vi "Curtin_CheckNewLoc.vi"(6 "Settings":T2={"Name of test"="", "Date"=timestamp(0 s since 1904-01-01), "Location"="", "Template"="", "Soundcard"="", "resolution"=32, "Sampling rate"=48000, "Ch1 Gain "=25.0, "Ch2 Gain"=10.0, "Sample time (s)"=0.3, "Pre-trigger (s)"=0.01, "Hammer Threshold"=10.0, "Positions"=12, "Taps/Position"=5, "Set Names"="", "Freq resolution"=10.0, "Hammer cutoff"=0.0, "Mic cutoff"=0.0, "Double bounce "=0.0, "Hammer Cal"=10.0, "dB Offset"=0.0, "Accel Cal"=10.0, "Vibrometer Cal"=0.0, "Mic Cal"=0.0, "Output"=2, "Voltage Cal"=1.0, "Vibrometer Port"="ASRL27::INSTR", "Range"=4, "High Pass"=2, "Bandwidth"=4, "X Range"=[], "Y Range"=[], "dB Spread"=0.0, "Trigger"=0, "Ch_1"=25, "Ch_2"=25, "flip?"=FALSE, "60Hz"=FALSE, "Time offset"=0.0, "Piezo Cal"=1.0, "Default Notes"=""} {"Ch_2" min=1 step=1; "Ch_1" min=1 max=100 step=1; "Trigger" items=["Hammer (force)", "Self-tap", "Spacebar"]; "Bandwidth" items=["1 kHz"=1, "5 kHz"=5, "10 kHz"=10, "25 kHz"=25, "50 kHz"=50, "100 kHz"=100]; "High Pass" items=["Off", "13 Hz", "104 Hz"]; "Range" items=["10 mm/s"=1, "20 mm/s"=2, "50 mm/s"=5, "100 mm/s"=10, "200 mm/s"=20, "500 mm/s"=50, "1 m/s"=100, "2 m/s"=200]; "Output" items=["Accelerometer", "Speed (from acceleration)", "Microphone", "Vibrometer", "Piezo"]; "Voltage Cal" format="%#_13g"; "Ch2 Gain" format="%#_13g"; "Ch1 Gain" format="%#_13g"; "Double bounce" min=0.0; "Mic cutoff" min=0.0 format="%#_4g"; "Hammer cutoff" min=0.0 format="%#_4g"; "Freq resolution" min=0.0; "Pre-trigger (s)" format="%#_13g"; "Date" format="%<%H:%M\n%d/%m/%y>T"; "resolution" items=["16 bit"=16, "24 bit"=24, "32 bit"=32]; "Sampling rate" items=["22050 samp/s"=22050, "44100 samp/s"=44100, "48000 samp/s"=48000]}, 8 "Last Data File":path, 11 "Alarms":refnum<vi>) -> (0 "Last Data Set":path, 1 "Task":T1(ring), 2 "Keep Set?":bool, 3 "Done?":bool, 4 "New Set":bool, 5 "Pause?":bool)   [LabVIEW 2022 SP3]
uses:
  PreferencesControl.ctl
  Mic_Global.vi
panel:
  # "Hz"
  # "dB"
  # "dB"
  # "sec"
  # "sec"
  # "mV/Pa"
  # "mV/m/s2"
  # "mV/mm/s"
  # "V/N"
  # "sec"
  # "sec"
  # "mV/N"
  # "a.u."
  # "a.u."
  # "sec"
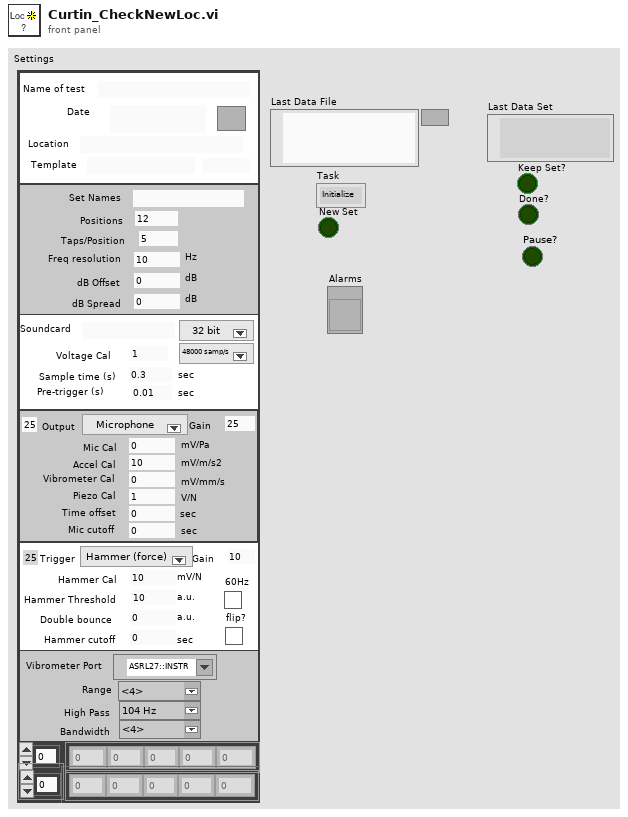
[diagram p1: front panel]
types:
  T1 = enum16{"Initialize", "Free run", "One Shot - waiting", "One Shot - triggered", "Wait", "Close"}
  T2 = typedef "PreferencesControl.ctl" = cluster{"Name of test":string, "Date":timestamp, "Location":string, "Template":string, "Soundcard":string, "resolution":u16, "Sampling rate":u16, "Ch1 Gain ":dbl, "Ch2 Gain":dbl, "Sample time (s)":dbl, "Pre-trigger (s)":dbl, "Hammer Threshold":dbl, "Positions":i16, "Taps/Position":i16, "Set Names":string, "Freq resolution":dbl, "Hammer cutoff":dbl, "Mic cutoff":dbl, "Double bounce ":dbl, "Hammer Cal":dbl, "dB Offset":dbl, "Accel Cal":dbl, "Vibrometer Cal":dbl, "Mic Cal":dbl, "Output":u16, "Voltage Cal":dbl, "Vibrometer Port":refnum<visa-resource-name>, "Range":u16, "High Pass":u16, "Bandwidth":u16, "X Range":cluster{"Minimum":dbl, "Maximum":dbl, "Increment":dbl, "Minor Increment":dbl, "Start":dbl}[], "Y Range":cluster{"Minimum":dbl, "Maximum":dbl, "Increment":dbl, "Minor Increment":dbl, "Start":dbl}[], "dB Spread":dbl, "Trigger":u16, "Ch_1":u8, "Ch_2":u8, "flip?":bool, "60Hz":bool, "Time offset":dbl, "Piezo Cal":dbl, "Default Notes":string}
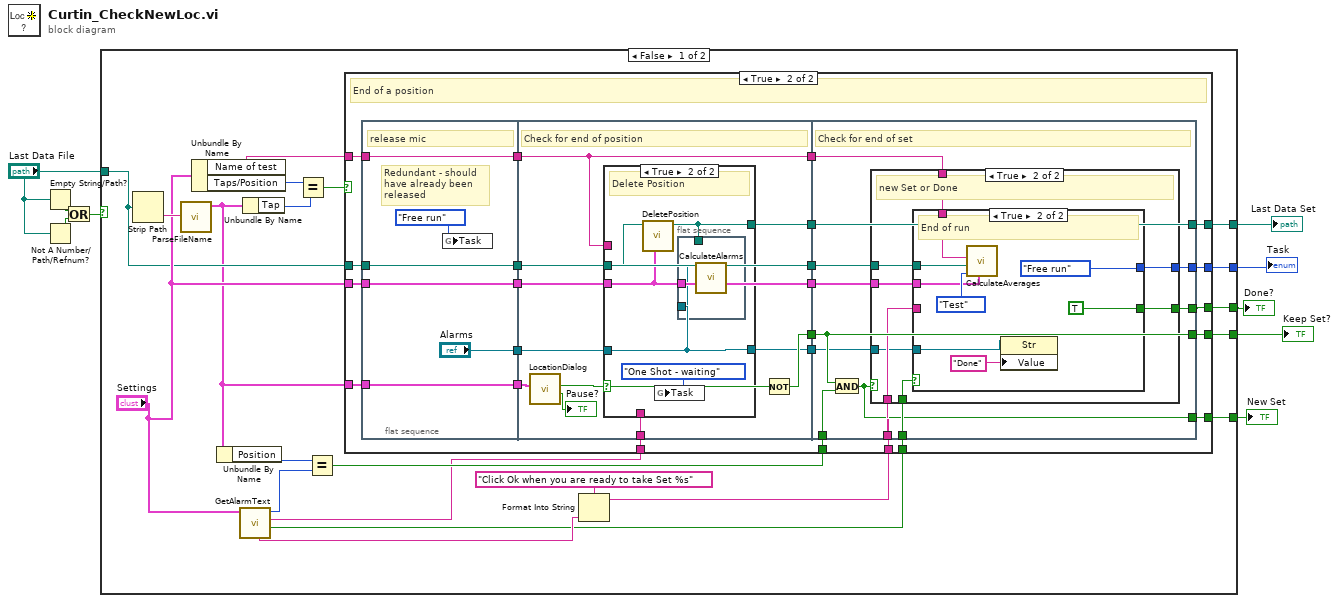
[diagram p0: block diagram]
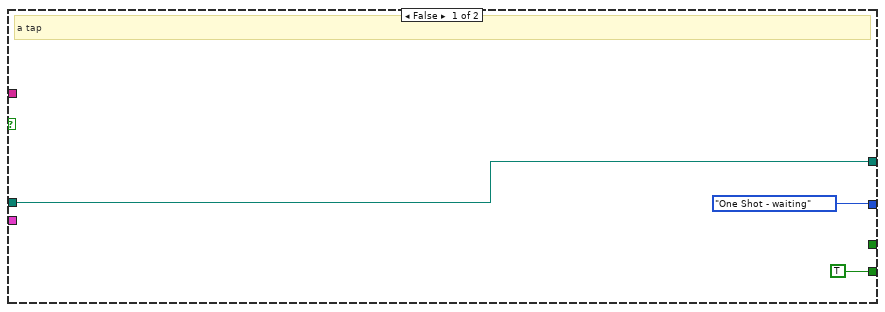
[diagram p2: hidden frame]
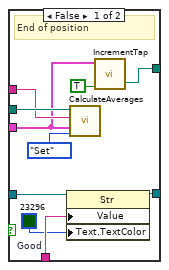
[diagram p3: hidden frame]
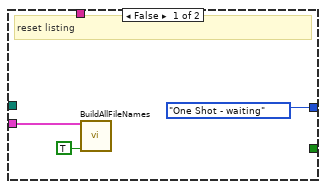
[diagram p4: hidden frame]
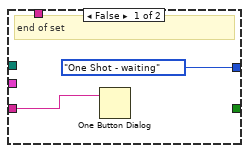
[diagram p5: hidden frame]
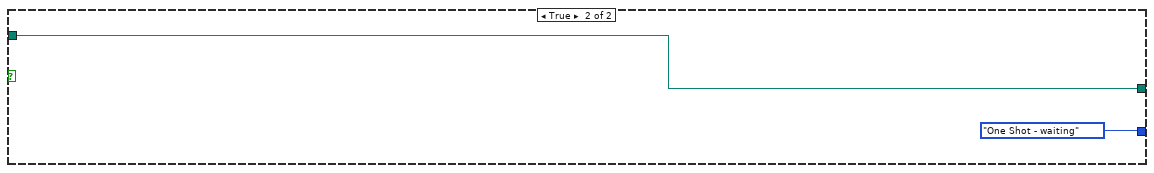
[diagram p6: hidden frame]
diagram:
  n1 = Empty String/Path?(string/path="Last Data File") -> (empty?=w5:bool)
  n2 = Not A Number/Path/Refnum?(number/path/refnum="Last Data File") -> (NaN/Path/Refnum?=w4:bool)
  n3 = Or(x=w5, y=w4) -> (x .or. y?=w3:bool)
  n4 = case shown="False" w3 {
    tunnel: [w23 _] -> w9
    tunnel: [w18 w126] -> w8
    tunnel: [w17 _] -> w7
    tunnel: "Last Data File" -> [w16 w126]
    tunnel: [w14 T1."One Shot - waiting" ("Task")] -> w2
    tunnel: [w13 _] -> w1
    frame False {
      n5 = Strip Path(path=w16) -> (name=w30:string)  [unwired: 1 out]
      n6 = call "ParseFileName.vi"("String in"=w30) -> ("Info"=w15:cluster{"Set":string, "Position":i32, "Tap":i32})  [unwired: 2 out]
      n7 = Unbundle By Name("Settings") -> ("Name of test"=w24:string, "Taps/Position"=w28:i16)
      n8 = Unbundle By Name(w15) -> ("Position"=w26:i32)
      n9 = call "GetAlarmText.vi"("Settings"="Settings") -> ("Done?"=w11:bool, "text"=w10:string, "Positions"=w27:i16, "Set Names"=w12:string)  [unwired: 7 in]
      n10 = Unbundle By Name(w15) -> ("Tap"=w29:i32)
      n11 = Equal?(x=w28, y=w29) -> (x = y?=w21:bool)
      n12 = Equal?(x=w26, y=w27) -> (x = y?=w25:bool)
      n13 = Format Into String(format string="Click Ok when you are ready to take Set %s" ("Text"), w12) -> (resulting string=w19:string)  [unwired: 2 in, 1 out]
      n14 = case shown="True" w21 {
        tunnel: w16 -> [w33 w57]
        tunnel: w19 -> [_ w55]
        tunnel: w25 -> [_ w54]
        tunnel: w11 -> [_ w53]
        tunnel: w24 -> [_ w45]
        tunnel: [_ w50] -> w23
        tunnel: "Settings" -> [_ w49]
        tunnel: [w33 w43] -> w18
        tunnel: [TRUE w41] -> w17
        tunnel: w15 -> [_ w40]
        tunnel: [T1."One Shot - waiting" ("Task") w38] -> w14
        tunnel: [_ w37] -> w13
        tunnel: w10 -> [_ w34]
        frame False {
          # "a tap"
        }
        frame True {
          # "End of a position"
          n15 = flat-sequence {
            tunnel: w57 -> [w62]
            tunnel: [w62] -> w56
            tunnel: w49 -> [w61]
            tunnel: [w61] -> w48
            tunnel: [w60] -> w46
            tunnel: w45 -> [w60]
            tunnel: w40 -> [w59]
            tunnel: [w59] -> w39
            tunnel: ["Alarms"] -> w36
            tunnel: w56 -> [w73]
            tunnel: [w69] -> w52
            tunnel: [w73] -> w51
            tunnel: w48 -> [w72]
            tunnel: [w72] -> w47
            tunnel: w46 -> [w71]
            tunnel: [w71] -> w44
            tunnel: [w70] -> w42
            tunnel: w39 -> [w68]
            tunnel: w36 -> [w67]
            tunnel: [w66] -> w35
            tunnel: w34 -> [w65]
            tunnel: w53 -> [w102]
            tunnel: w54 -> [w101]
            tunnel: w55 -> [w103]
            tunnel: w52 -> [w95]
            tunnel: w51 -> [w100]
            tunnel: [w99] -> w50
            tunnel: w47 -> [w98]
            tunnel: w44 -> [w97]
            tunnel: [w96] -> w43
            tunnel: w42 -> [w96]
            tunnel: [w95] -> w41
            tunnel: [w94] -> w38
            tunnel: [w93] -> w37
            tunnel: w35 -> [w92]
            frame #0 {
              # "Redundant - should\nhave already been\nreleased"
              # "release mic"
              n16 = global write "Mic_Global.vi" "Task"(T1."Free run" ("Task")) -> ()
            }
            frame #1 {
              # "Check for end of position"
              n17 = call "LocationDialog.vi"("Info"=w68) -> ("Pause?"=→"Pause?":bool, "Redo?"=w74:bool)  [unwired: 9 in]
              n18 = case shown="True" w74 {
                tunnel: w73 -> [w84 w89]
                tunnel: [w77 w86] -> w70
                tunnel: w71 -> [w82 _]
                tunnel: w72 -> [w80 w85]
                tunnel: w67 -> [w79 w87]
                tunnel: [w76 w87] -> w66
                tunnel: w65 -> [w78 _]
                frame False {
                  w75 = u32 23296  # Good
                  # "End of position"
                  n19 = property class="Str"(reference=w79, "Value"=w78, "Text.TextColor"=w75) -> (reference out=w76:refnum<vi>)  [unwired: 1 in, 1 out]
                  n20 = call "CalculateAverages.vi"("Settings"=w80, "Task"=enum16{"Set", "Test"}."Set", "Inst:Test Name"=w82, "Last Data File"=w84) -> ()  [unwired: 8 in]
                  n21 = call "IncrementTap.vi"("Reset?"=TRUE, "Settings"=w80) -> ("Last Data Set"=w77:path)  [unwired: 4 in, 5 out]
                }
                frame True {
                  # "Delete Position"
                  n22 = call "DeletePosition.vi"("Settings"=w85, "last"=w89) -> ("Last Data Set"=w86:path)  [unwired: 8 in, 1 out]
                  n23 = global write "Mic_Global.vi" "Task"(T1."One Shot - waiting" ("Task")) -> ()
                  n24 = flat-sequence {
                    tunnel: w87 -> [w91]
                    tunnel: w85 -> [w90]
                    tunnel: w86 -> [_]
                    frame #0 {
                      n25 = call "CalculateAlarms.vi"("Settings"=w90, "Alarm"=w91) -> ()  [unwired: 8 in, 2 out]
                    }
                  }
                }
              }
              n26 = Not(x=w74) -> (.not. x?=w69:bool)
            }
            frame #2 {
              # "Check for end of set"
              n27 = And(x=w95, y=w101) -> (x .and. y?=w93:bool)
              n28 = case shown="True" w93 {
                tunnel: w103 -> [_ w113]
                tunnel: w102 -> [_ w114]
                tunnel: w100 -> [_ w112]
                tunnel: w97 -> [_ w111]
                tunnel: [_ w110] -> w99
                tunnel: w98 -> [w104 w109]
                tunnel: [T1."One Shot - waiting" ("Task") w108] -> w94
                tunnel: w92 -> [_ w107]
                frame False {
                  # "reset listing"
                  n29 = call "BuildAllFileNames.vi"("Reset?"=TRUE, "Settings"=w104) -> ()  [unwired: 8 in, 2 out]
                }
                frame True {
                  # "new Set or Done"
                  n30 = case shown="True" w114 {
                    tunnel: w113 -> [w116 _]
                    tunnel: [T1."One Shot - waiting" ("Task") T1."Free run" ("Task")] -> w108
                    tunnel: w112 -> [_ w123]
                    tunnel: w111 -> [_ w121]
                    tunnel: [_ TRUE] -> w110
                    tunnel: w109 -> [_ w119]
                    tunnel: w107 -> [_ w118]
                    frame False {
                      # "end of set"
                      n31 = One Button Dialog(message=w116) -> ()  [unwired: 1 in, 1 out]
                    }
                    frame True {
                      # "End of run"
                      n32 = call "CalculateAverages.vi"("Settings"=w119, "Task"=enum16{"Set", "Test"}."Test", "Inst:Test Name"=w121, "Last Data File"=w123) -> ()  [unwired: 8 in]
                      n33 = property class="Str"(reference=w118, "Value"="Done") -> ()  [unwired: 1 in, 2 out]
                    }
                  }
                }
              }
            }
          }
        }
      }
    }
    frame True {
    }
  }
  "Done?" <- w9
  "Last Data Set" <- w8
  "Keep Set?" <- w7
  "Task" <- w2
  "New Set" <- w1
